vi "rql_New Connection.vi"(4 "Show in Debugger?":bool=TRUE, 6 "Message Priority":T1=enum."Normal", 8 "error in":errorcluster, 10 "Data in":T2, 11 "TCP Client in":refnum<class "TCP Client.lvclass">) -> (0 "error out":errorcluster, 3 "dup TCP Client out":refnum<class "TCP Client.lvclass">)   [LabVIEW 2017, in "TCP Client.lvlib" / "TCP Client.lvclass"]
doc: "This VI sends a <b>Local API Request</b> message to an MHL case of the Worker that owns this VI.\n---\nA new TCP connection has been established with a TCP Server."
uses:
  TCP Client.lvclass
  C:/Program Files (x86)/National Instruments/LabVIEW 2017/vi.lib/addons/_Workers/Library/Classes/Worker/Worker.lvclass
  rql_New Connection.ctl
  <vilib>/addons/_Workers/Library/Classes/Message/Priority.ctl
  <vilib>/addons/_Workers/Library/Case Label.ctl
  <vilib>/addons/_Workers/Library/Classes/Message Queue/Message Queue.lvclass
  <vilib>/addons/_Workers/Library/Workers.lvlib
  <vilib>/addons/_Workers/Library/Classes/Message/Message.lvclass
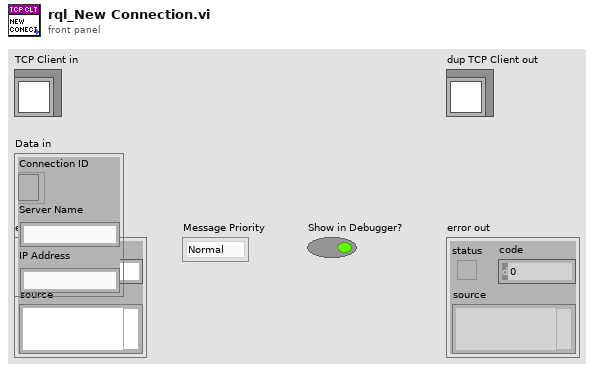
[diagram p1: front panel]
types:
  T1 = typedef "Workers.lvlib/Message.lvclass/Priority.ctl" = enum16{"Low", "Normal", "High"}
  T2 = typedef "TCP Client.lvlib/TCP Client.lvclass/rql_New Connection.ctl" = cluster{"Connection ID":refnum<k5>, "Server Name":string, "IP Address":string}
  T3 = typedef "Workers.lvlib/Case Label.ctl" = string
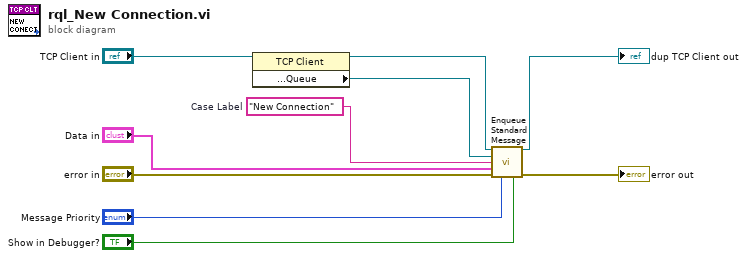
[diagram p0: block diagram]
diagram:
  w1 = T3 "New Connection"  # Case Label
  n1 = property class="TCP Client"(reference="TCP Client in") -> (reference out=w3:refnum<class "TCP Client.lvclass">, "Accessors:Read:Public API:Queue"=w2:refnum<class "Message Queue.lvclass">)  [unwired: 1 in, 1 out]
  n2 = call-dynamic "Enqueue Standard Message.vi"("Worker"=w3, "Message Queue"=w2, "Case Label"=w1, "Data"="Data in", "error in (no error)"="error in", "Priority (Normal)"="Message Priority", "Send Message to Debugger? (T)"="Show in Debugger?") -> ("dup Worker out"=→"dup TCP Client out":refnum<class "TCP Client.lvclass">, "error out"=→"error out":errorcluster)  [unwired: 7 in]
